vi "Create Message Metadata.vi"(8 "error in (no error)":errorcluster, 11 "ProtoFile Messages":u64[](array[numeric])) -> (0 "error out":errorcluster, 3 "Message Parameters":T1[](array[typedef]))   [LabVIEW 2019, in "gRPC Template Creation Utility.lvlib"]
uses:
  gRPC Template Creation Utility.lvlib
  TypeDefs/Message Metadata (Scripting).ctl
  TypeDefs/Message Element Metadata (Scripting).ctl
  TypeDefs/Message Element Type.ctl
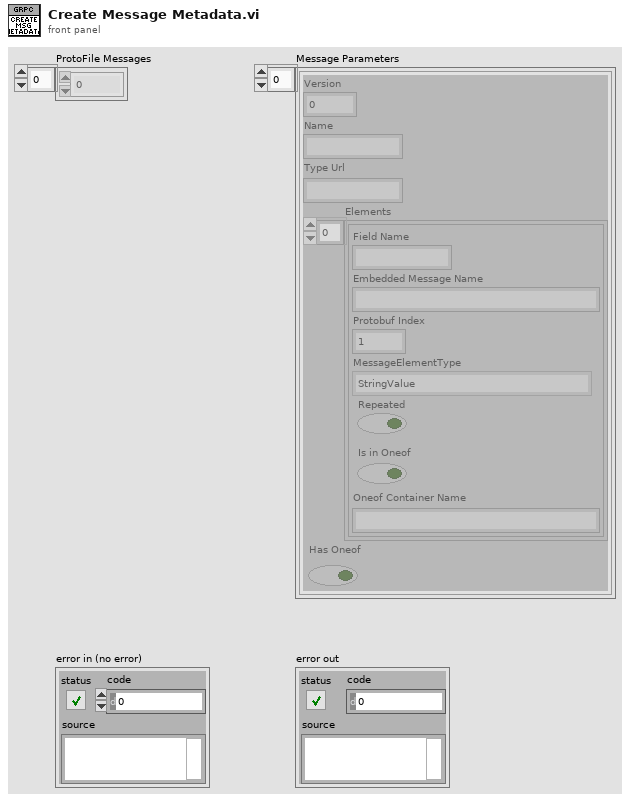
[diagram p1: front panel]
types:
  T1 = typedef "gRPC Template Creation Utility.lvlib/Message Metadata (Scripting).ctl" = cluster{"Version":i32, "Name":string, "Type Url":string, "Elements":T2[], "Has Oneof":bool}
  T2 = typedef "gRPC Template Creation Utility.lvlib/Message Element Metadata (Scripting).ctl" = cluster{"Field Name":string, "Embedded Message Name":string, "Protobuf Index":i32, "MessageElementType":T3, "Repeated":bool, "Is in Oneof":bool, "Oneof Container Name":string}
  T3 = typedef "gRPC Template Creation Utility.lvlib/Message Element Type.ctl" = enum32{"Int32Value", "FloatValue", "DoubleValue", "BoolValue", "StringValue", "MessageValue", "Int64Value", "UInt32Value", "UInt64Value", "EnumValue", "Bytes", "Fixed64", "Fixed32", "SFixed64", "SFixed32", "SInt64", "SInt32"}
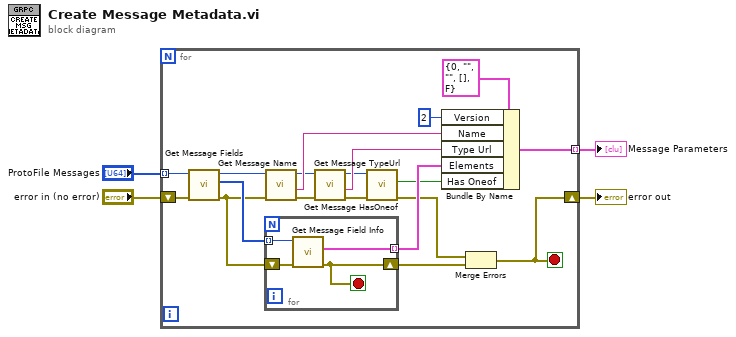
[diagram p0: block diagram]
diagram:
  n1 = for {
    tunnel: "ProtoFile Messages" -> [w23] mode=indexing
    shift-right: [w16] -> w3
    shift-left: "error in (no error)" -> [w20]
    tunnel: [w17] -> w1 mode=indexing
    stop <- w16 stop-if-true
    n2 = call "Get Message Fields.vi"("error in (no error)"=w20, "Message ref in"=w23) -> ("error out"=w19:errorcluster, "Field refs"=w22:u64[], "Message ref out"=w10:u64)  [unwired: 7 in]
    n3 = for {
      tunnel: w22 -> [w27] mode=indexing
      tunnel: [w26] -> w14 mode=indexing
      shift-right: [w24] -> w18
      shift-left: w19 -> [w25]
      stop <- w24 stop-if-true
      n4 = call "Get Message Field Info.vi"("error in (no error)"=w25, "Message Field ref in"=w27) -> ("error out"=w24:errorcluster, "Field Info"=w26:T2)  [unwired: 7 in, 1 out]
    }
    n5 = call "Get Message Name.vi"("error in (no error)"=w19, "Message ref in"=w10) -> ("error out"=w13:errorcluster, "Message Name"=w15:string, "Message ref out"=w6:u64)  [unwired: 7 in]
    n6 = call "Get Message TypeUrl.vi"("error in (no error)"=w13, "Message ref in"=w6) -> ("error out"=w9:errorcluster, "Message Name"=w12:string, "Message ref out"=w5:u64)  [unwired: 7 in]
    n7 = call "Get Message HasOneof.vi"("error in (no error)"=w9, "Message ref in"=w5) -> ("error out"=w8:errorcluster, "Has Oneof?"=w7:bool)  [unwired: 7 in, 1 out]
    n8 = Bundle By Name(cluster=T1 {"Version"=0, "Name"="", "Type Url"="", "Elements"=[], "Has Oneof"=FALSE} ("Message Metadata"), "Version"=2, "Name"=w15, "Type Url"=w12, "Elements"=w14, "Has Oneof"=w7) -> (w17:T1)
    n9 = Merge Errors(w8, w18) -> (w16:errorcluster)
  }
  "Message Parameters" <- w1
  "error out" <- w3
